vi "CR-字符检测处理函数.vi"(8 "error in (no error)":errorcluster caption="错误输入（无错误）", 10 "CR- 字符检测参数":T2={"Threshold Data"={"Method"=enum."Local", "Looking for"=1, "Color Mode"=0, "Kernel Size"={"Width"=32, "Height"=32}, "Ranges"=[{"Min"=1, "Max"=255}]}, "Reject Border"=TRUE, "Number Of Erosions"=0, "Size & Spacing"={"Segment Algorithm"=0, "Min Bounding Rect Width"=1, "Max Bounding Rect Width"=65536, "Min Bounding Rect Height"=1, "Max Bounding Rect Height"=65536, "Min Character Size"=20, "Max Character Size"=65536, "Min Char Spacing"=1, "Max Horiz Element Spacing"=1, "Max Vert Element Spacing"=0, "Max Space Distance"=65536}, "Read Options"={"Read Strategy"=1, "Read Resolution"=2, "Scale Dependant"=FALSE, "Aspect Ratio"=400, "Acceptance Level"=700, "Substitution Character"="?", "MultiLine"=TRUE}, "Valid Characters"=[], "Use Text Pattern"=FALSE, "Orientation"=0, "# Lines Expected"=0, "Number of Blocks"=4, "Rectangle"={"Left"=0, "Top"=0, "Right"=0, "Bottom"=0, "Rotation"=0.0}, "File Path (字符库)"=path "D:/Inspect System/Source Code/Template Program/字符模板.abc", "Url"="http://10.6.1.31:8080/MesInnerpackLineIO.asmx。", "accessKey"="a45b2d3334ffs_\n", "字符长度设定"=0, "File Path (连接件模板)"=path "D:/Inspect System/Source Code/Template Program/字符检测定位模板.png"} {"Rectangle"."Rotation" min=-90.0 max=90.0 step=1.0 format="%.2f"; "Rectangle"."Left" scale=0.0..1024.0; "Rectangle"."Right" scale=0.0..1024.0; "Threshold Data"."Looking for" items=["Light on Dark", "Dark on Light"]; "Threshold Data"."Color Mode" items=["RGB", "HSL", "HSV", "HSI"]; "Size & Spacing"."Segment Algorithm" items=["None", "Shortest Segment", "Legacy Auto Split"]; "Read Options"."Read Strategy" items=["Aggressive", "Conservative"]; "Read Options"."Read Resolution" items=["Low", "Medium", "High"]; "Valid Characters"."Pre-defined characters" items=["Any Character", "User-defined Characters", "Alphabetic", "Alphanumeric", "Uppercase Letters", "Lowercase Letters", "Decimal Digits", "Hexadecimal Digits", "Pattern", "Force Space"]; "Orientation" items=["Baseline inside", "Baseline outside"]}, 11 "Image in":T3(plugin-control)) -> (0 "error out":errorcluster caption="错误输出", 1 "布尔":bool, 2 "String (OCR/OCV 1)":string, 3 "Image out":T3(plugin-control), 4 "匹配后偏移量":i32)   [LabVIEW 2017]
panel:
  in  "Advanced Options (Pattern Matching 1)":cluster{"Item":u16, "Value":dbl}[](array[cluster])=[{"Item"=102, "Value"=10.0}, {"Item"=106, "Value"=300.0}, {"Item"=107, "Value"=0.0}, {"Item"=108, "Value"=6.0}, {"Item"=109, "Value"=1.0}, {"Item"=114, "Value"=25.0}, {"Item"=111, "Value"=20.0}, {"Item"=112, "Value"=10.0}, {"Item"=113, "Value"=20.0}, {"Item"=103, "Value"=1.0}, {"Item"=104, "Value"=20.0}, {"Item"=105, "Value"=0.0}, {"Item"=100, "Value"=6.0}] {"Item" items=["LD Sampling - Minimum Constrast"=0, "LD Sampling - Enable Subpixel Accuracy"=1, "LD Sampling - Search Strategy"=2, "LD Sampling - Subpixel Iterations"=3, "LD Sampling - Subpixel Tolerance"=4, "LD Sampling - Initial Match List Length"=5, "LD Sampling - Match List Reduction Factor"=6, "LD Sampling - Initial Step Size"=7, "LD Sampling - Intermediate Angular Accuracy"=8, "-"=9, "Pyramid - Max Pyramid Level"=100, "Pyramid - Minimum Contrast"=102, "Pyramid - Enable Subpixel Accuracy"=103, "Pyramid - Subpixel Iterations"=104, "Pyramid - Subpixel Tolerance"=105, "Pyramid - Initial Match List Length"=106, "Pyramid - Match List Reduction Factor"=107, "Pyramid - Intermediate Angular Accuracy"=108, "Pyramid - Process Border Matches"=109, "Pyramid - Min Match Separation Distance"=111, "Pyramid - Min Match Separation Angle"=112, "Pyramid - Max Match Overlap"=113, "Pyramid - Max Cache in MB"=114, "Pyramid - Clear Cache"=115, "-"=116, "Enable Defect Map"=200]}
  out "长度":i32
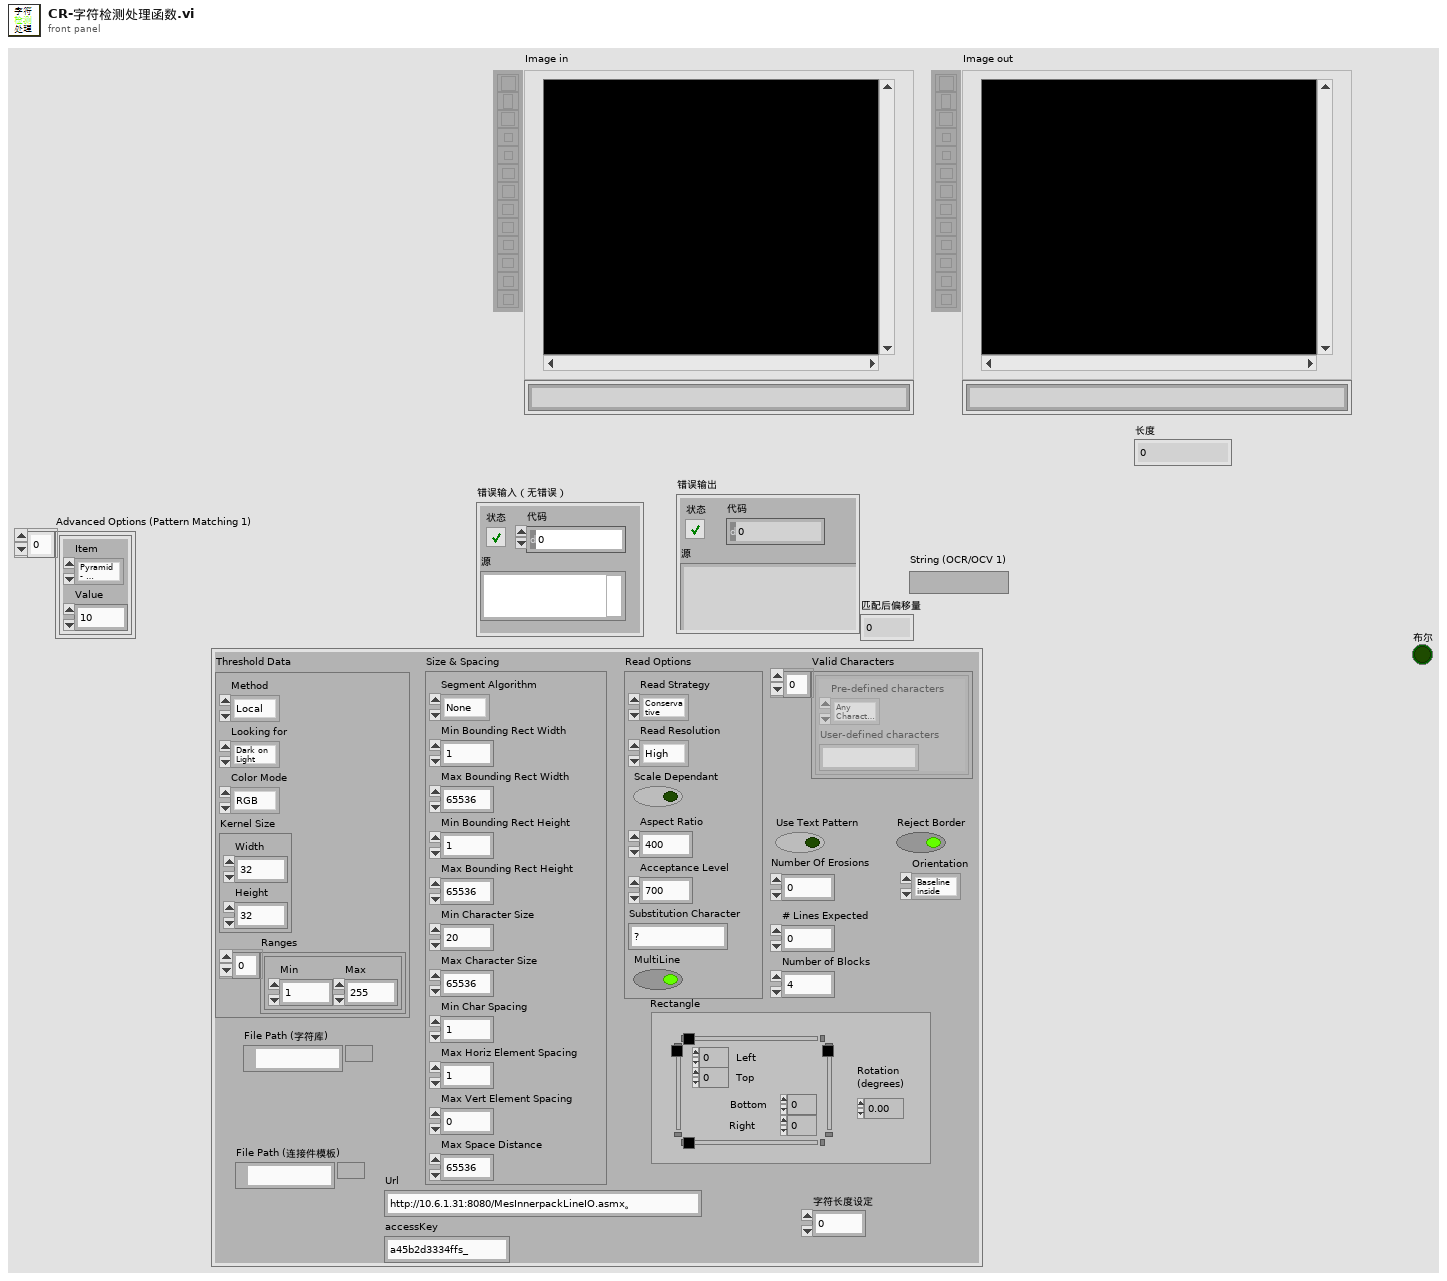
[diagram p1: front panel]
types:
  T1 = typedef "IMAQ Rectangle" = cluster{"Left":i32, "Top":i32, "Right":i32, "Bottom":i32, "Rotation":dbl}
  T2 = cluster{"Threshold Data":cluster{"Method":enum16{"Fixed Range", "Uniform", "Linear", "Non Linear", "Local", "Color"}, "Looking for":u32, "Color Mode":u32, "Kernel Size":cluster{"Width":i32, "Height":i32}, "Ranges":cluster{"Min":i32, "Max":i32}[]}, "Reject Border":bool, "Number Of Erosions":i32, "Size & Spacing":cluster{"Segment Algorithm":u16, "Min Bounding Rect Width":i32, "Max Bounding Rect Width":i32, "Min Bounding Rect Height":i32, "Max Bounding Rect Height":i32, "Min Character Size":i32, "Max Character Size":i32, "Min Char Spacing":i32, "Max Horiz Element Spacing":i32, "Max Vert Element Spacing":i32, "Max Space Distance":i32}, "Read Options":cluster{"Read Strategy":i32, "Read Resolution":i32, "Scale Dependant":bool, "Aspect Ratio":i32, "Acceptance Level":i32, "Substitution Character":string, "MultiLine":bool}, "Valid Characters":cluster{"Pre-defined characters":i32, "User-defined characters":string}[], "Use Text Pattern":bool, "Orientation":u32, "# Lines Expected":u32, "Number of Blocks":i32, "Rectangle":T1, "File Path (字符库)":path, "Url":string, "accessKey":string, "字符长度设定":i32, "File Path (连接件模板)":path}
  T3 = typedef "IMAQ Image.ctl" = refnum<image>
  T4 = cluster{"Global Rectangle":i32[], "Contours":cluster{"ID":enum32{"External", "Internal"}, "Type":u32, "Coordinates":i32[]}[]}
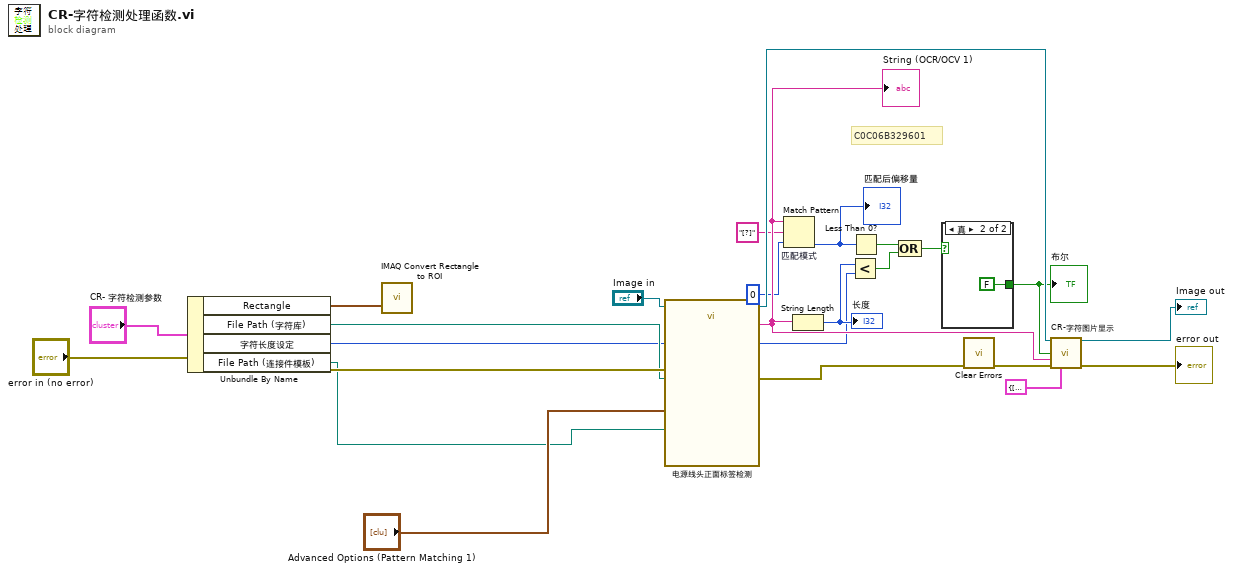
[diagram p0: block diagram]
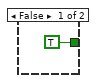
[diagram p2: hidden frame]
diagram:
  # "C0C06B329601"
  n1 = Unbundle By Name("CR- 字符检测参数") -> ("Rectangle"=w4:T1, "File Path (字符库)"=w10:path, "字符长度设定"=w3:i32, "File Path (连接件模板)"=w1:path)
  n2 = call "IMAQ Convert Rectangle to ROI"("Rectangle"=w4) -> ()  [unwired: 8 in, 2 out]
  n3 = call "电源线头正面标签检测"("Image In"="Image in", "Advanced Options (Pattern Matching 1)"="Advanced Options (Pattern Matching 1)", "Template File Path (Pattern Matching 1)"=w1, "error in"="error in (no error)", "File Path (OCR/OCV 1)"=w10) -> ("Image Out"=w21:T3, "String (OCR/OCV 1)"=w9:string, "error out"=w17:errorcluster)  [unwired: 18 in, 2 out]
  "String (OCR/OCV 1)" <- w9
  n4 = Match Pattern "匹配模式"(string=w9, regular expression="[?]" ("格式字符串"), offset (0)=0 ("偏移量(0)")) -> (offset past match=w6:i32)  [unwired: 3 out]
  "匹配后偏移量" <- w6
  n5 = String Length(string=w9) -> (length=w15:i32)
  "长度" <- w15
  n6 = Less?(x=w15, y=w3) -> (x < y?=w12:bool)
  n7 = Less Than 0?(x=w6) -> (x < 0?=w5:bool)
  n8 = Compound Arithmetic op=OR ("复合运算")(w5, w12) -> (w11:bool)
  n9 = case shown="真" w11 {
    tunnel: [TRUE FALSE] -> w16
    frame False {
    }
    frame True {
    }
  }
  "布尔" <- w16
  n10 = call <vilib>:"Clear Errors.vi"("error in (no error)"=w17) -> ("error out"=w18:errorcluster)  [unwired: 5 in, 1 out]
  n11 = call "CR-字符图片显示.vi"("Image in"=w21, "是否检测到字符串"=w16, "String (OCR/OCV 1)"=w9, "error in (no error)"=w18, "ROI Descriptor"=T4 {"Global Rectangle"=[733, 718, 1751, 851], "Contours"=[{"ID"=enum."External", "Type"=12, "Coordinates"=[734, 727, 1750, 842, 988]}]} ("ROI Descriptor (OCR/OCV 1)")) -> ("Image out"=→"Image out":T3, "error out"=→"error out":errorcluster)  [unwired: 9 in]
